vi "Clear Limit Failure.vi"(8 "error in (no error)":errorcluster, 10 "Calculate Block (1: Calculate Block 1)":i32(ring)=1 items=["Calculate Block 1"=1, "Calculate Block 2"=2, "Calculate Block 3"=3, "Calculate Block 4"=4], 11 "VISA resource name":refnum<visa-resource-name>) -> (0 "error out":errorcluster, 3 "VISA resource name out":refnum<visa-resource-name>)   [LabVIEW 2018, in "Agilent U2000 Series.lvlib"]
doc: "Performs clearance of FCO (fail counter)."
uses:
  Agilent U2000 Series.lvlib
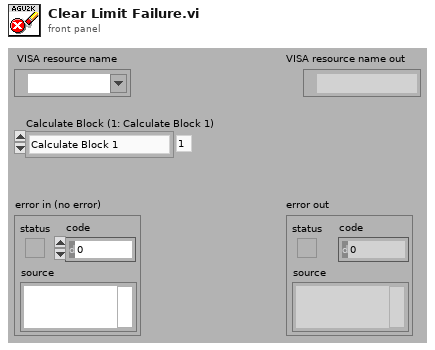
[diagram p1: front panel]
types:
  T1 = typedef "Agilent U2000 Series.lvlib/Extended User Data.ctl" = cluster{"U2000 Series Mode":u16, "Trigger Source Int/Ext":bool}
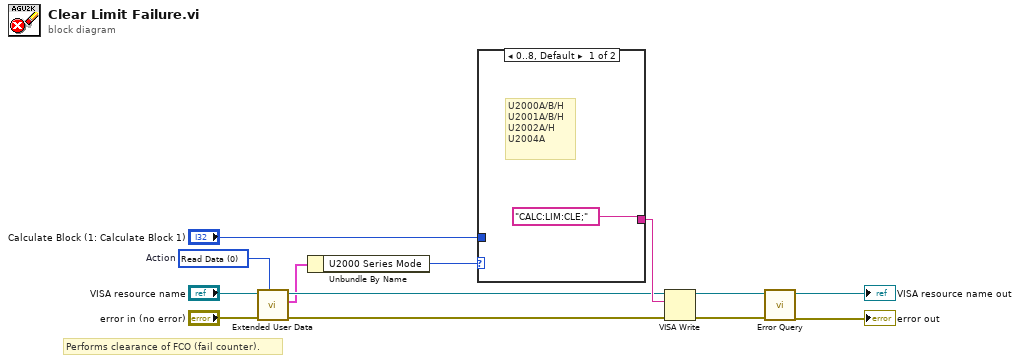
[diagram p0: block diagram]
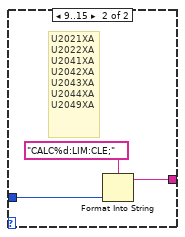
[diagram p2: hidden frame]
diagram:
  w1 = 0 items=["Read Data", "Write Data", "Clear Data", "Clear ALL Data"]  # Action
  # "Performs clearance of FCO (fail counter)."
  n1 = call "Extended User Data.vi"("Action (1: Write Data)"=w1, "error in (no error)"="error in (no error)", "VISA resource name"="VISA resource name") -> ("error out"=w5:errorcluster, "User Data Out"=w3:T1, "VISA resource name out"=w4:refnum<visa-resource-name>)  [unwired: 1 in, 5 out]
  n2 = Unbundle By Name(w3) -> ("U2000 Series Mode"=w2:u16)
  n3 = case shown="0..8, Default" w2 {
    tunnel: "Calculate Block (1: Calculate Block 1)" -> [_ w17]
    tunnel: ["CALC:LIM:CLE;" w15] -> w8
    frame 0..8, Default {
      # "U2000A/B/H\nU2001A/B/H\nU2002A/H\nU2004A"
    }
    frame 9..15 {
      # "U2021XA\nU2022XA\nU2041XA\nU2042XA\nU2043XA\nU2044XA\nU2049XA"
      n4 = Format Into String(format string="CALC%d:LIM:CLE;", w17) -> (resulting string=w15:string)  [unwired: 2 in, 1 out]
    }
  }
  n5 = VISA Write(VISA resource name=w4, write buffer=w8, error in (no error)=w5) -> (VISA resource name out=w13:refnum<visa-resource-name>, error out=w12:errorcluster)  [unwired: 1 out]
  n6 = call "Error Query.vi"("error in (no error)"=w12, "VISA resource name"=w13) -> ("error out"=→"error out":errorcluster, "VISA resource name out"=→"VISA resource name out":refnum<visa-resource-name>)  [unwired: 8 out]
